vi "UDP - Receiver.vi"(8 "error in (no error)":errorcluster, 11 "UDP Ports to Check":u16[](array[numeric])=[44525, 44515]) -> (0 "error out":errorcluster, 2 "log file path":path, 3 "Results":string[][](array[string]))   [LabVIEW 2019]
doc: "The UDP protocol differs from TCP in that there is no error-checking with the packets of information that are sent, and thus no guarantee whatsoever that an intended recipient will actually receive a given piece of data.\n\nUDP does offer the ability to \"broadcast\" data across a network--simply specify an IP Address of all ones (255.255.255.255) to attempt to broadcast information network-wide. Keep in mind that routers and other network hardware will generally refuse to forward the broadcast beyond certain points, so the extent of the broadcast will in practice be limited."
panel:
  out "log file name":string
  out "Current test":cluster{string, "error out":errorcluster}
  out "current port":u16
  in  "Start test":bool
  out "Received Data":dbl(graph)
  # "Overview: Listens for data from UDP - Sender.vi on ports in UDP Ports to Check array. Returns received data in graphical and array form and logs the results to disc.\n\nInstructions:\n1. Ensure UDP - Sender.vi is already running.\n2. Run the VI.\n3. Click Start to start the test."
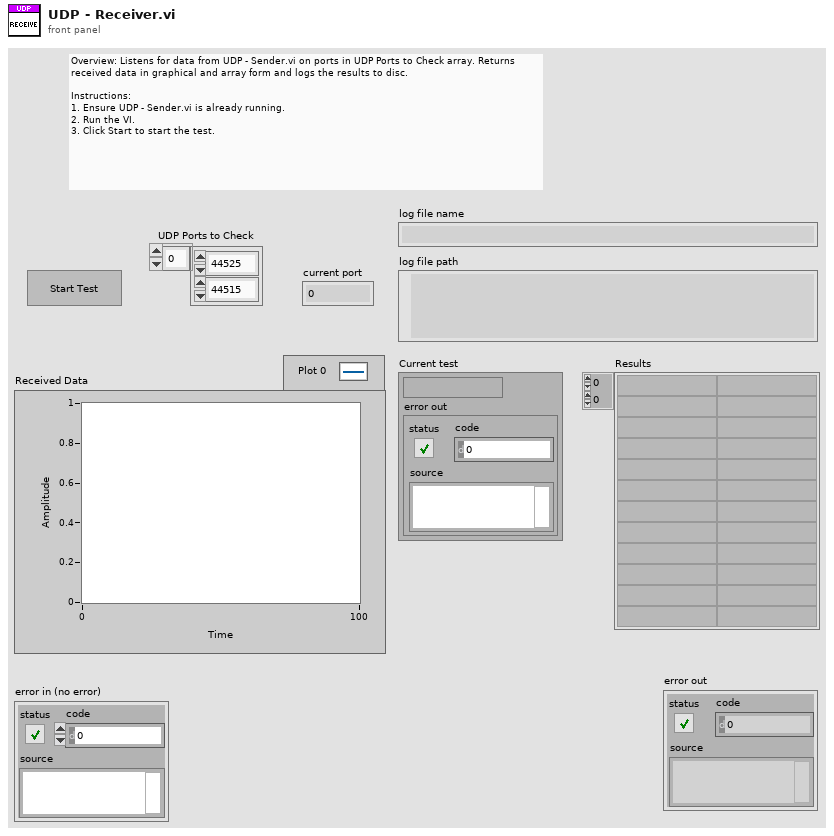
[diagram p1: front panel]
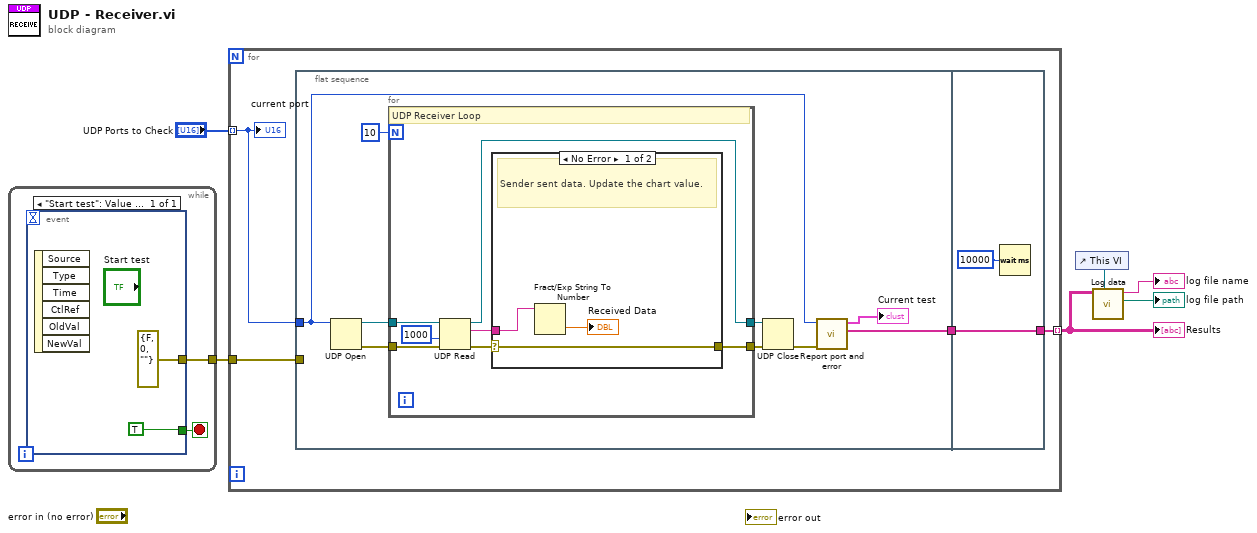
[diagram p0: block diagram]
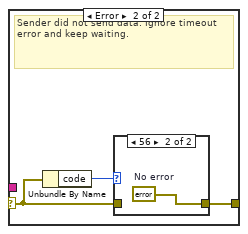
[diagram p2: hidden frame]
diagram:
  n1 = while {
    tunnel: [w8] -> w5
    stop <- w7 stop-if-true
    n2 = event shown="[0] \"Start test\": Value Change" {
      selector: _ -> [_]
      dyn-events: _ -> [_]
      timeout: _ -> [_]
      tunnel: [errorcluster {"status"=FALSE, "code"=0, "source"=""} ("error constant")] -> w8
      tunnel: [TRUE] -> w7
      event "Start test": Value Change {
        n3 = event-data() -> ()  [unwired: 1 in, 6 out]
      }
    }
  }
  n4 = for {
    tunnel: "UDP Ports to Check" -> [w14] mode=indexing
    tunnel: w5 -> [w12]
    tunnel: [w11] -> w1 mode=indexing
    n5 = flat-sequence {
      tunnel: w14 -> [w17]
      tunnel: [w15] -> w13
      tunnel: w12 -> [_]
      tunnel: w13 -> [w39]
      tunnel: [w39] -> w11
      frame #0 {
        n6 = UDP Open(11:w17) -> (port=w20:refnum<k16>, 0:w21:errorcluster)  [unwired: 4 in, 1 out]
        n7 = for {
          N: 10 -> [_]
          tunnel: w20 -> [w30]
          tunnel: [w24] -> w23
          tunnel: w21 -> [w29]
          tunnel: [w25] -> w22
          # "UDP Receiver Loop"
          n8 = UDP Read(connection ID=w30, timeout ms (25000)=1000, 8:w29) -> (data out=w27:string, error out=w26:errorcluster, 3:w24:refnum<k16>)  [unwired: 3 out]
          n9 = case shown="No Error" w26 {
            selector: w26 -> [w31 w35]
            tunnel: w27 -> [w33 _]
            tunnel: [w31 w34] -> w25
            frame No Error {
              # "Sender sent data. Update the chart value."
              n10 = Fract/Exp String To Number(string=w33) -> (number=→"Received Data":dbl)  [unwired: 3 in, 1 out]
            }
            frame Error {
              # "Sender did not send data. Ignore timeout error and keep waiting."
              n11 = Unbundle By Name(w35) -> ("code"=w36:i32)
              n12 = case shown="56" w36 {
                tunnel: w35 -> [w37 _]
                tunnel: [w37 w38] -> w34
                frame Default {
                }
                frame 56 {
                  w38 = errorcluster {"status"=FALSE, "code"=0, "source"=""}  # No error
                }
              }
            }
          }
        }
        n13 = UDP Close(connection ID=w23, 8:w22) -> (error out=w16:errorcluster)  [unwired: 1 out]
        n14 = call "Report port and error.vi"("error in (no error)"=w16, "port"=w17) -> ("Array"=w15:string[], "output cluster"=→"Current test":cluster{string, "error out":errorcluster})  [unwired: 7 in, 1 out]
      }
      frame #1 {
        n15 = Wait (ms)(milliseconds to wait=u32 10000) -> ()  [unwired: 1 out]
      }
    }
    "current port" <- w14
  }
  "Results" <- w1
  n16 = control-ref of="This VI"() -> (w2:refnum<vi>)
  n17 = call "Log data.vi"(7:w2, 11:w1) -> ("log file path"=→"log file path":path, "log file name"=→"log file name":string)  [unwired: 7 in, 1 out]
